vi "Run Macro.vi"(8 "error in (no error)":errorcluster, 10 "Macro Name":string, 11 "Motions in":refnum<class "Motions.lvclass">) -> (0 "error out":errorcluster, 3 "Motions out":refnum<class "Motions.lvclass">)   [LabVIEW 2016, in "Hardware.lvlib" / "Motions.lvlib" / "Motions.lvclass"]
uses:
  <userlib>/Common Components/Hardware/Abstract System/Motions/Motions/Motions.lvclass
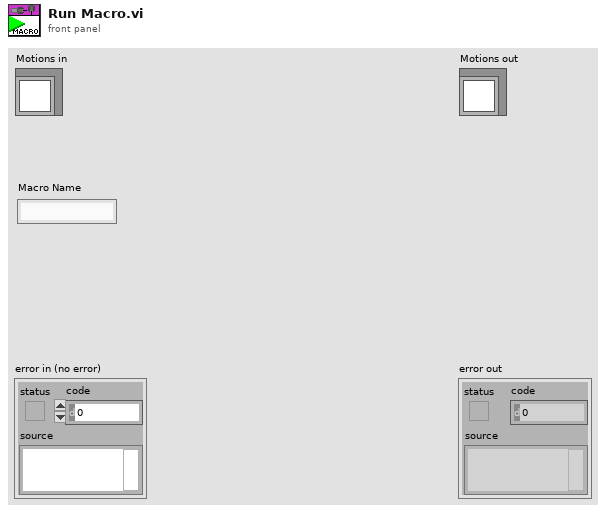
[diagram p1: front panel]
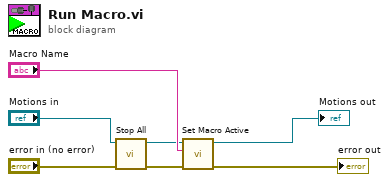
[diagram p0: block diagram]
diagram:
  n1 = call <userlib>:"Stop All.vi"("error in (no error)"="error in (no error)", "Motions in"="Motions in") -> ("error out"=w3:errorcluster, "Motions out"=w1:refnum<class "Motions.lvclass">)  [unwired: 8 in]
  n2 = call <userlib>:"Set Macro Active.vi"("error in (no error)"=w3, "Macro Name"="Macro Name", "Motions in"=w1) -> ("error out"=→"error out":errorcluster, "Motions out"=→"Motions out":refnum<class "Motions.lvclass">)  [unwired: 7 in]
